vi "DeferCallerPanel.vi"(2 "On/Off":bool, 5 "Dispose":bool, 7 "error in (no error)":errorcluster) -> (6 "error out":errorcluster)   [LabVIEW 2020, in "CameraTestingUI.lvlib" / "CameraTestingUI.lvclass"]
uses:
  CameraTestingUI.lvclass
  CameraTestingUI.lvclass/CameraTestingUI.ctl
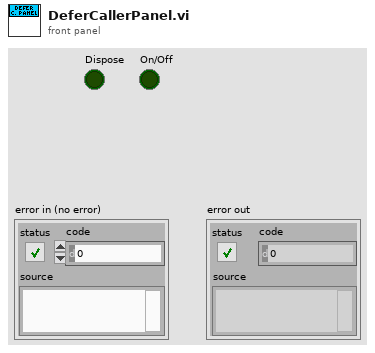
[diagram p1: front panel]
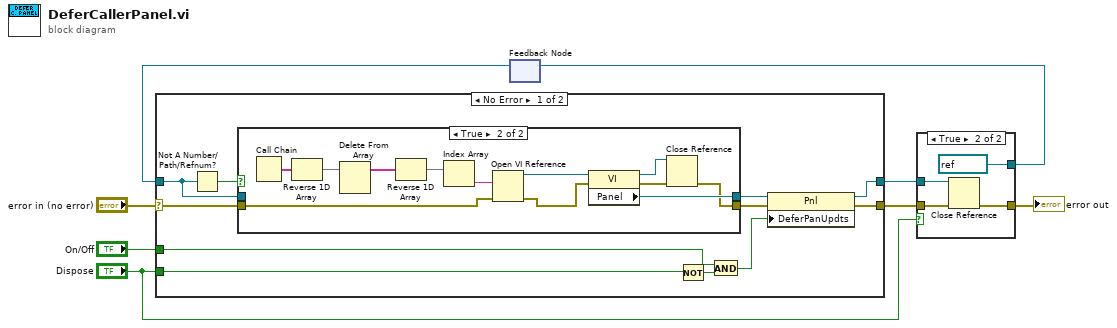
[diagram p0: block diagram]
diagram:
  n1 = feedback #1() -> (w6:refnum<vi>)  [unwired: 1 in]
  n2 = case shown="No Error" "error in (no error)" {
    selector: "error in (no error)" -> [w18 w35]
    tunnel: [w17 w35] -> w5
    tunnel: "On/Off" -> [w10 _]
    tunnel: [w14 w34] -> w3
    tunnel: w6 -> [w13 w34]
    tunnel: "Dispose" -> [w12 _]
    frame No Error {
      n3 = Not A Number/Path/Refnum?(number/path/refnum=w13) -> (NaN/Path/Refnum?=w15:bool)
      n4 = case shown="True" w15 {
        tunnel: [w21 w32] -> w16
        tunnel: [w20 w28] -> w19
        tunnel: w18 -> [w20 w27]
        tunnel: w13 -> [w21 _]
        frame False {
        }
        frame True {
          n5 = Call Chain() -> (call chain=w25:string[])
          n6 = Reverse 1D Array(array=w25) -> (reversed array=w26:string[])
          n7 = Delete From Array(array=w26) -> (array with subset deleted=w24:string[])  [unwired: 2 in, 1 out]
          n8 = Reverse 1D Array(array=w24) -> (reversed array=w23:string[])
          n9 = Index Array(array=w23) -> (element=w22:string)  [unwired: 1 in]
          n10 = Open VI Reference(vi path=w22, error in (no error)=w27) -> (vi reference=w33:refnum<vi>, error out=w31:errorcluster)  [unwired: 4 in]
          n11 = property class="VI"(reference=w33, error in=w31) -> (reference out=w29:refnum<vi>, error out=w30:errorcluster, "Panel"=w32:refnum<vi>)
          n12 = Close Reference(reference=w29, error in (no error)=w30) -> (error out=w28:errorcluster)
        }
      }
      n13 = Not(x=w12) -> (.not. x?=w11:bool)
      n14 = And(x=w10, y=w11) -> (x .and. y?=w9:bool)
      n15 = property class="Pnl"(reference=w16, error in=w19, "DeferPanUpdts"=w9) -> (reference out=w14:refnum<vi>, error out=w17:errorcluster)
    }
    frame Error {
    }
  }
  n16 = case shown="True" "Dispose" {
    tunnel: w5 -> [w37 w41]
    tunnel: w3 -> [w36 w40]
    tunnel: [w37 w39] -> w2
    tunnel: [w36 refnum<vi> refnum ("Panel")] -> w1
    frame False {
    }
    frame True {
      n17 = Close Reference(reference=w40, error in (no error)=w41) -> (error out=w39:errorcluster)
    }
  }
  "error out" <- w2
  n18 = feedback-in #1(w1) -> ()
